vi "Custom Aggregation (DBL).vi"(0 "data in":dbl, 1 "reset? (F)":bool, 5 "aggregation settings":T1={"interval"=1, "interval unit"=enum."Runs", "synchronization of intervals"=enum."Not synchronized", "algorithm"=enum."Average"}, 9 "system info in":refnum<class "EP System Info.lvclass">, 11 "error in (no error)":errorcluster, 12 "data timestamp":timestamp) -> (4 "aggregated minimum value":dbl, 6 "aggregated averaged/RMS value":dbl, 8 "aggregated maximum value":dbl, 10 "system info out":refnum<class "EP System Info.lvclass">, 13 "aggregated data valid?":bool, 14 "aggregated data timestamp":timestamp, 15 "error out":errorcluster)   [LabVIEW 2014, in "NI_EP_Power Quality.lvlib"]
doc: "Calculates the aggregated minimum, maximum, and averaged or RMS value of an input signal for a specified aggregation interval, according to Class S in IEC 61000-4-30:2008. There is no overlap between aggregation intervals. This VI automatically restarts accumulation at the beginning of the next time interval after the previous interval expires. You must manually select the polymorphic instance you want to use.\n\nThis VI supports measuring single-line and multiple-line systems except the DBL instance. Use the DBL instance to measure one channel on one line at one time."
uses:
  <vilib>/addons/Electrical Power/PQ/NI_EP_Power Quality.lvlib
  <vilib>/addons/Electrical Power/PQ/Common/Controls/ep_Aggregation Settings.ctl
  <vilib>/addons/Electrical Power/PQ/Common/Classes/System Info/EP System Info.lvclass
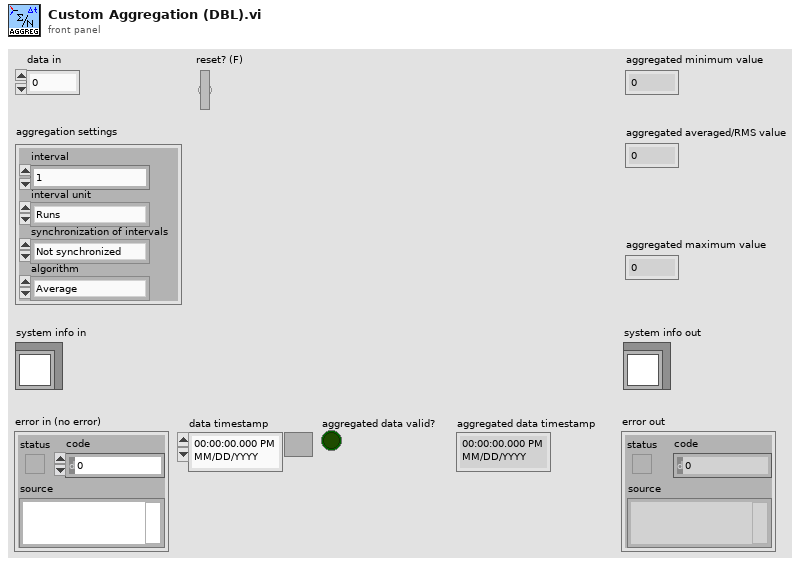
[diagram p1: front panel]
types:
  T1 = typedef "NI_EP_Power Quality.lvlib/ep_Aggregation Settings.ctl" = cluster{"interval":u32, "interval unit":enum16{"Runs", "Seconds", "Minutes", "Hours", "Days", "Weeks"}, "synchronization of intervals":enum16{"Not synchronized", "Interval rounded"}, "algorithm":enum16{"Average", "RMS"}}
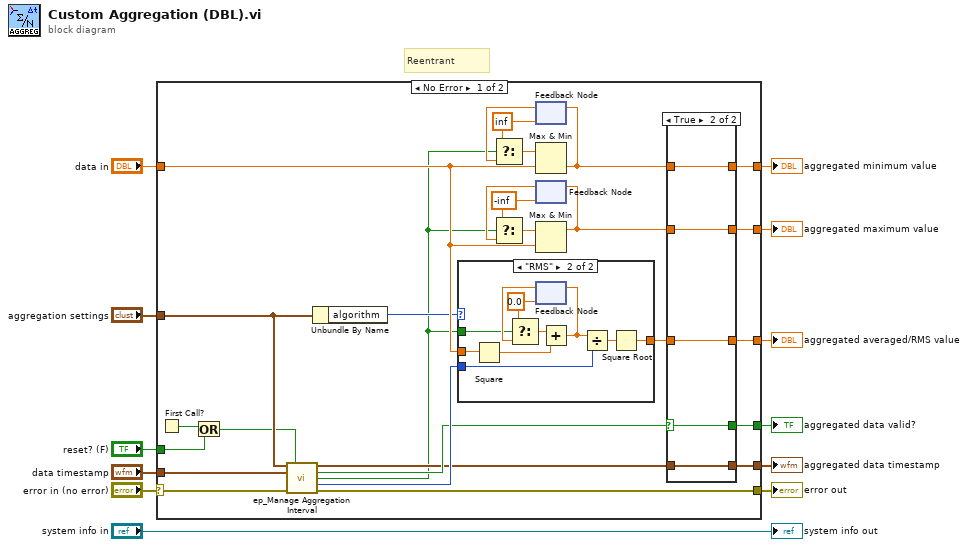
[diagram p0: block diagram]
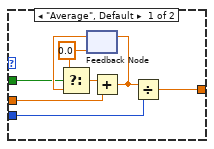
[diagram p3: hidden frame]
diagram:
  # "Reentrant"
  n1 = case shown="No Error" "error in (no error)" {
    selector: "error in (no error)" -> [w19 w64]
    tunnel: "reset? (F)" -> [w14 _]
    tunnel: "data in" -> [w33 _]
    tunnel: "aggregation settings" -> [w16 _]
    tunnel: "data timestamp" -> [w31 _]
    tunnel: [w29 w64] -> w8
    tunnel: [w18 _] -> w7
    tunnel: [w27 _] -> w6
    tunnel: [w23 _] -> w5
    tunnel: [w22 _] -> w4
    tunnel: [w20 _] -> w3
    frame No Error {
      w34 = -inf
      w39 = inf
      n2 = First Call?() -> (First Call?: T/F=w15:bool)
      n3 = Or(x=w15, y=w14) -> (x .or. y?=w13:bool)
      n4 = call <vilib>:"ep_Manage Aggregation Interval.vi"("aggregation settings"=w16, "restart (F)"=w13, "data time stamp"=w31, "error in (no error)"=w19) -> ("aggregated data time stamp"=w21:timestamp, "aggregated data valid?"=w28:bool, "restart aggregation?"=w17:bool, "runs"=w30:u32, "error out"=w29:errorcluster)  [unwired: 7 in]
      n5 = Unbundle By Name(w16) -> ("algorithm"=w32:enum16{"Average", "RMS"})
      n6 = case shown="\"RMS\"" w32 {
        tunnel: w33 -> [w47 w57]
        tunnel: w17 -> [w48 w58]
        tunnel: w30 -> [w53 w63]
        tunnel: [w52 w54] -> w26
        frame "Average", Default {
          w50 = 0.0
          n7 = feedback #1(w50) -> (w51:dbl)
          n8 = Select(t=w50, s=w48, f=w51) -> (s? t:f=w49:dbl)
          n9 = Add(x=w49, y=w47) -> (x+y=w46:dbl)
          n10 = feedback-in #1(w46) -> ()
          n11 = Divide(x=w46, y=w53) -> (x/y=w52:dbl)
        }
        frame "RMS" {
          w60 = 0.0
          n12 = Square(x=w57) -> (x^2=w55:dbl)
          n13 = feedback #2(w60) -> (w61:dbl)
          n14 = Select(t=w60, s=w58, f=w61) -> (s? t:f=w59:dbl)
          n15 = Add(x=w59, y=w55) -> (x+y=w56:dbl)
          n16 = feedback-in #2(w56) -> ()
          n17 = Divide(x=w56, y=w63) -> (x/y=w62:dbl)
          n18 = Square Root(x=w62) -> (sqrt(x)=w54:dbl)
        }
      }
      n19 = feedback #3(w39) -> (w38:dbl)
      n20 = Select(t=w39, s=w17, f=w38) -> (s? t:f=w37:dbl)
      n21 = Max & Min(x=w37, y=w33) -> (min(x,y)=w24:dbl)  [unwired: 1 out]
      n22 = feedback-in #3(w24) -> ()
      n23 = feedback #4(w34) -> (w35:dbl)
      n24 = Select(t=w34, s=w17, f=w35) -> (s? t:f=w36:dbl)
      n25 = Max & Min(x=w36, y=w33) -> (max(x,y)=w25:dbl)  [unwired: 1 out]
      n26 = feedback-in #4(w25) -> ()
      n27 = case shown="True" w28 {
        selector: w28 -> [w40 w41]
        tunnel: [_ w45] -> w27
        tunnel: w26 -> [_ w45]
        tunnel: w25 -> [_ w43]
        tunnel: w24 -> [_ w44]
        tunnel: [_ w44] -> w23
        tunnel: [_ w43] -> w22
        tunnel: w21 -> [_ w42]
        tunnel: [_ w42] -> w20
        tunnel: [w40 w41] -> w18
        frame False {
        }
        frame True {
        }
      }
    }
    frame Error {
    }
  }
  "error out" <- w8
  "aggregated minimum value" <- w5
  "aggregated averaged/RMS value" <- w6
  "aggregated maximum value" <- w4
  "aggregated data valid?" <- w7
  "aggregated data timestamp" <- w3
  "system info out" <- "system info in"
